vi "CloseMetodo.vi"(8 "error in (no error)":errorcluster, 11 "Keysight in":refnum<class "Edu-1200.lvclass">) -> (0 "error out":errorcluster, 3 "Keysight out":refnum<class "Edu-1200.lvclass">)   [LabVIEW 2020, in "Edu-1200.lvclass"]
uses:
  Edu-1200.lvclass
  Edu-1200.lvclass/Edu-1200.ctl
  <instrlib>/Agilent 2000 3000 X-Series/Agilent 2000 3000 X-Series.lvlib
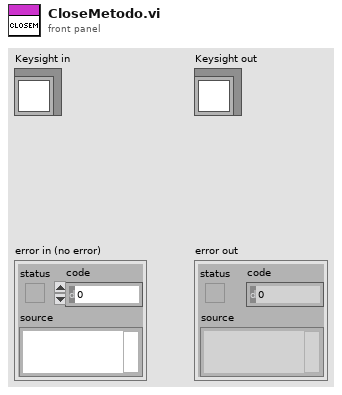
[diagram p1: front panel]
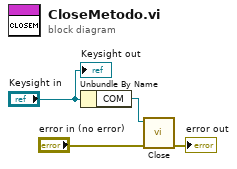
[diagram p0: block diagram]
diagram:
  n1 = Unbundle By Name("Keysight in") -> ("COM"=w3:refnum<visa-resource-name>)
  n2 = call <instrlib>:"Close.vi"("error in (no error)"="error in (no error)", "VISA resource name"=w3) -> ("error out"=→"error out":errorcluster)  [unwired: 9 in]
  "Keysight out" <- "Keysight in"
